vi "Compare VS Config to Database Changes.vi"(8 "error in (no error)":errorcluster, 9 "VS Existing Frames":T3[](array[typedef]) {"Node Ref" format="%.0x"}, 10 "Old Cluster":refnum<k21>, 11 "New Cluster":refnum<k21>) -> (0 "error out":errorcluster, 3 "Database Changes":T1 {"Missing"."Node Ref" format="%.0x"; "Changed"."Old"."Node Ref" format="%.0x"})   [LabVIEW 2025, in "Protection and Counter Addon System Explorer.lvlib"]
uses:
  Protection and Counter Addon System Explorer.lvlib
  Types/Base Frame Info.ctl
  <vilib>/NI VeriStand/Custom Device API/Custom Device Item Ref.ctl
  Types/Database Changes.ctl
  Types/Base Frame Info_NoVS.ctl
  Types/Related CAN Frames.ctl
  Types/Related CAN Frames No VS.ctl
  <vilib>/NI VeriStand/Custom Device API/Custom Device API.lvlib
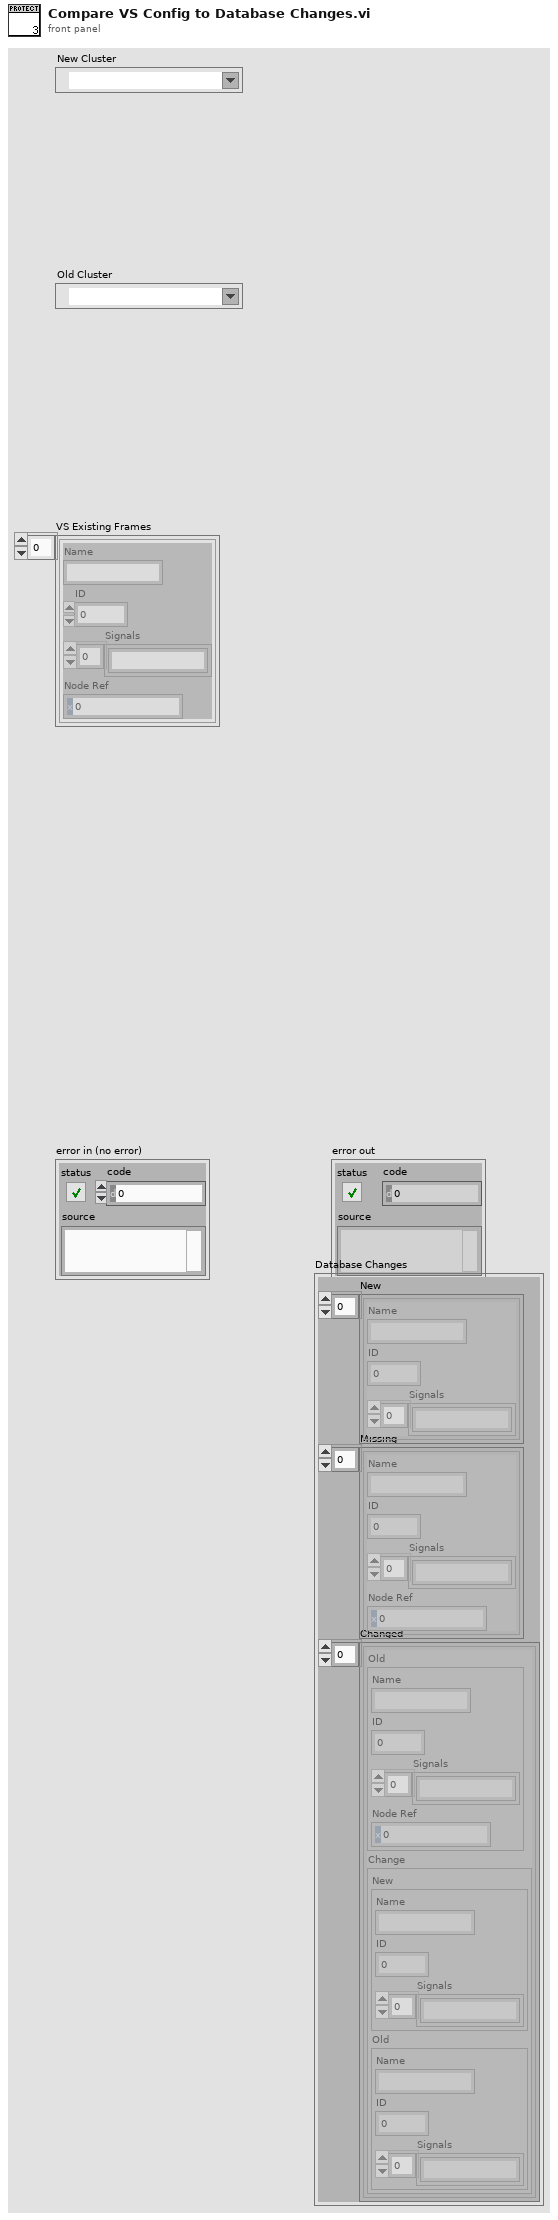
[diagram p1: front panel]
types:
  T1 = typedef "Protection and Counter Addon System Explorer.lvlib/Database Changes.ctl" = cluster{"New":T2[], "Missing":T3[], "Changed":T5[]}
  T2 = typedef "Protection and Counter Addon System Explorer.lvlib/Base Frame Info_NoVS.ctl" = cluster{"Name":string, "ID":u32, "Signals":string[]}
  T3 = typedef "Protection and Counter Addon System Explorer.lvlib/Base Frame Info.ctl" = cluster{"Name":string, "ID":u32, "Signals":string[], "Node Ref":T4}
  T4 = typedef "Custom Device API.lvlib/Custom Device Item Ref.ctl" = u64
  T5 = typedef "Protection and Counter Addon System Explorer.lvlib/Related CAN Frames.ctl" = cluster{"Old":T3, "Change":T6}
  T6 = typedef "Protection and Counter Addon System Explorer.lvlib/Related CAN Frames No VS.ctl" = cluster{"New":T2, "Old":T2}
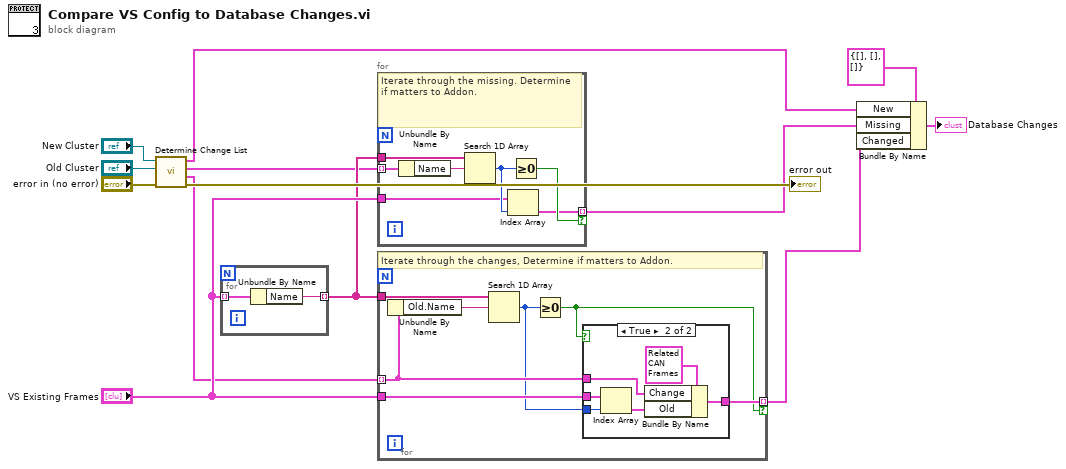
[diagram p0: block diagram]
diagram:
  n1 = call "Determine Change List.vi"("error in (no error)"="error in (no error)", "Old Cluster"="Old Cluster", "New Cluster"="New Cluster") -> ("error out"=→"error out":errorcluster, "Changed"=w6:T6[], "Missing"=w7:T2[], "New"=w5:T2[])  [unwired: 5 in]
  n2 = for {
    tunnel: "VS Existing Frames" -> [w15] mode=indexing
    tunnel: [w14] -> w8 mode=indexing
    n3 = Unbundle By Name(w15) -> ("Name"=w14:string)
  }
  n4 = for {
    tunnel: w7 -> [w21] mode=indexing
    tunnel: w8 -> [w20]
    tunnel: [w16] -> w4 mode=indexing if=w19
    tunnel: "VS Existing Frames" -> [w17]
    # "Iterate through the missing. Determine if matters to Addon."
    n5 = Unbundle By Name(w21) -> ("Name"=w22:string)
    n6 = Search 1D Array(1D array=w20, element=w22) -> (index of element=w18:i32)  [unwired: 1 in]
    n7 = Index Array(array=w17, index=w18) -> (element=w16:T3)
    n8 = Greater Or Equal To 0?(x=w18) -> (x >= 0?=w19:bool)
  }
  n9 = for {
    tunnel: w6 -> [w25] mode=indexing
    tunnel: w8 -> [w28]
    tunnel: "VS Existing Frames" -> [w27]
    tunnel: [w26] -> w3 mode=indexing if=w24
    # "Iterate through the changes, Determine if matters to Addon."
    n10 = Unbundle By Name(w25) -> ("Old.Name"=w29:string)
    n11 = Search 1D Array(1D array=w28, element=w29) -> (index of element=w23:i32)  [unwired: 1 in]
    n12 = Greater Or Equal To 0?(x=w23) -> (x >= 0?=w24:bool)
    n13 = case shown="True" w24 {
      tunnel: w27 -> [_ w35]
      tunnel: w23 -> [_ w34]
      tunnel: [_ w33] -> w26
      tunnel: w25 -> [_ w32]
      frame False {
      }
      frame True {
        n14 = Index Array(array=w35, index=w34) -> (element=w30:T3)
        n15 = Bundle By Name(cluster=T5 {"Old"={"Name"="", "ID"=0, "Signals"=[], "Node Ref"=0}, "Change"={"New"={"Name"="", "ID"=0, "Signals"=[]}, "Old"={"Name"="", "ID"=0, "Signals"=[]}}}, "Change"=w32, "Old"=w30) -> (w33:T5)
      }
    }
  }
  n16 = Bundle By Name(cluster=T1 {"New"=[], "Missing"=[], "Changed"=[]}, "New"=w5, "Missing"=w4, "Changed"=w3) -> (→"Database Changes":T1)
